vi "CalcSeeds.vi"(2 "String":string) -> (6 "Seeds":cluster{"Start":i64, "End":i64}[](array[cluster]))   [LabVIEW 2022 SP3]
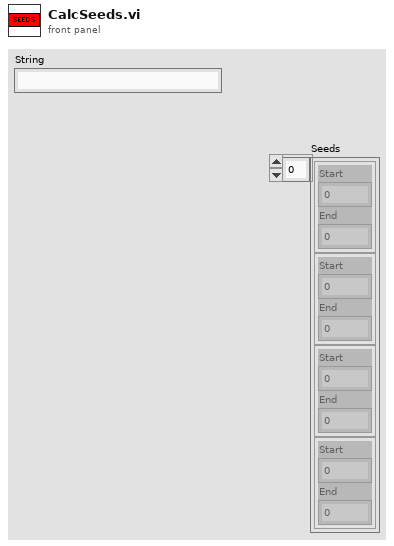
[diagram p1: front panel]
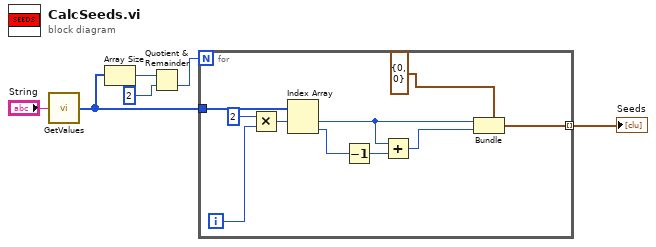
[diagram p0: block diagram]
diagram:
  n1 = call "GetValues.vi"("String"="String") -> ("Values"=w5:i64[])  [unwired: 6 in]
  n2 = Array Size(array=w5) -> (size(s)=w4:i32)
  n3 = Quotient & Remainder(x=w4, y=2) -> (floor(x/y)=w3:i32)  [unwired: 1 out]
  n4 = for {
    N: w3 -> [_]
    tunnel: w5 -> [w16]
    tunnel: [w12] -> w1 mode=indexing
    i -> [w15]
    n5 = Multiply(x=2, y=w15) -> (x*y=w14:i32)
    n6 = Index Array(array=w16, index #1=w14) -> (element #1=w9:i64, element #2=w11:i64)  [unwired: 1 in]
    n7 = Decrement(x=w11) -> (x-1=w10:i64)
    n8 = Add(x=w9, y=w10) -> (x+y=w8:i64)
    n9 = Bundle(cluster=cluster{"Start":i64, "End":i64} {"Start"=0, "End"=0} ("Source"), "Start"=w9, "End"=w8) -> (w12:cluster{"Start":i64, "End":i64})
  }
  "Seeds" <- w1
